vi "Debug - TCP - Log IP and Port.vi"(9 "IP and Port String":string, 10 "Flattened TCP Reference":string) -> ()   [LabVIEW 2017, in "Communications Library.lvlib"]
doc: "Edits the TCP debugging log file, so that the IP address and port are included in the contents.\n\nSaves changes to the file."
uses:
  Communications Library.lvlib
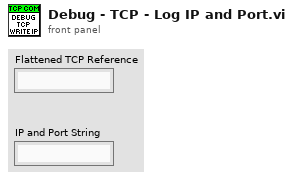
[diagram p1: front panel]
types:
  T1 = enum16{"open", "replace", "create", "open or create", "replace or create", "replace or create with confirmation"}
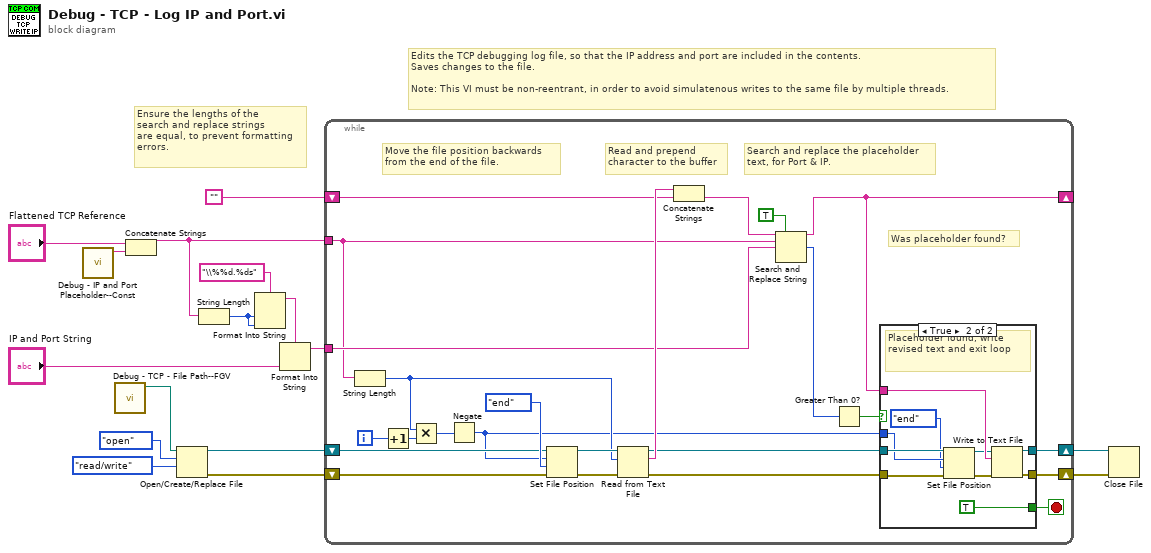
[diagram p0: block diagram]
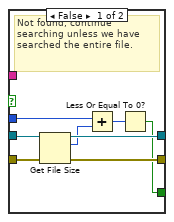
[diagram p2: hidden frame]
diagram:
  # "Ensure the lengths of the\nsearch and replace strings\nare equal, to prevent formatting\nerrors."
  # "Edits the TCP debugging log file, so that the IP address and port are included in the contents.\nSaves changes to the file.\n\nNote: This VI must be non-reentrant, in order to avoid simulatenous writes to the same file by multiple threads."
  n1 = call "Debug - IP and Port Placeholder--Const.vi"() -> ("Debug Placeholder"=w9:string)  [unwired: 11 in]
  n2 = call "Debug - TCP - File Path--FGV.vi"() -> ("Debug Pathname"=w7:path)  [unwired: 11 in]
  n3 = Concatenate Strings("Flattened TCP Reference", w9) -> (w3:string)
  n4 = Open/Create/Replace File(file path (use dialog)=w7, operation (0:open)=T1."open", access (0:read/write)=enum16{"read/write", "read-only", "write-only"}."read/write") -> (refnum out=w15:refnum<file>, error out=w16:errorcluster)  [unwired: 3 in, 1 out]
  n5 = String Length(string=w3) -> (length=w5:i32)
  n6 = Format Into String(format string="\\%%d.%ds", w5, w5) -> (resulting string=w6:string)  [unwired: 2 in, 1 out]
  n7 = Format Into String(format string=w6, "IP and Port String") -> (resulting string=w1:string)  [unwired: 2 in, 1 out]
  n8 = while {
    shift-right: [w18] -> _
    shift-left: "" -> [w30]
    tunnel: w3 -> [w17]
    tunnel: w1 -> [w28]
    shift-right: [w23] -> w10
    shift-left: w15 -> [w38]
    shift-right: [w22] -> w11
    shift-left: w16 -> [w39]
    i -> [w37]
    stop <- w21 stop-if-true
    # "Was placeholder found?"
    # "Search and replace the placeholder \ntext, for Port & IP."
    # "Read and prepend\ncharacter to the buffer"
    # "Move the file position backwards\nfrom the end of the file."
    n9 = String Length(string=w17) -> (length=w32:i32)
    n10 = Increment(x=w37) -> (x+1=w36:i32)
    n11 = Multiply(x=w32, y=w36) -> (x*y=w35:i32)
    n12 = Negate(x=w35) -> (-x=w20:i32)
    n13 = Set File Position(offset (in bytes) (0)=w20, refnum=w38, from (0:start)=enum16{"start", "end", "current"}."end", error in=w39) -> (refnum out=w34:refnum<file>, error out=w33:errorcluster)
    n14 = Read from Text File(file (use dialog)=w34, count=w32, error in=w33) -> (refnum out=w24:refnum<file>, text=w31:string, error out=w25:errorcluster)  [unwired: 1 in, 1 out]
    n15 = Concatenate Strings(w31, w30) -> (w19:string)
    n16 = Search and Replace String(replace all?=TRUE ("replace all? (F)"), input string=w19, search string=w17, replace string=w28) -> (result string=w18:string, number of replacements=w27:i32)  [unwired: 4 in, 2 out]
    n17 = Greater Than 0?(x=w27) -> (x > 0?=w26:bool)
    n18 = case shown="True" w26 {
      tunnel: w18 -> [_ w58]
      tunnel: w25 -> [w48 w54]
      tunnel: w24 -> [w47 w51]
      tunnel: [w46 w57] -> w23
      tunnel: [w45 w56] -> w22
      tunnel: [w41 TRUE] -> w21
      tunnel: w20 -> [w43 w50]
      frame False {
        # "Not found, continue\nsearching unless we have\nsearched the entire file."
        n19 = Get File Size(file=w47, error in=w48) -> (refnum out=w46:refnum<file>, size (in bytes)=w42:i64, 0:w45:errorcluster)
        n20 = Add(x=w43, y=w42) -> (x+y=w44:i64)
        n21 = Less Or Equal To 0?(x=w44) -> (x <= 0?=w41:bool)
      }
      frame True {
        # "Placeholder found, write\nrevised text and exit loop"
        n22 = Set File Position(offset (in bytes) (0)=w50, refnum=w51, from (0:start)=enum16{"start", "end", "current"}."end", error in=w54) -> (refnum out=w52:refnum<file>, error out=w53:errorcluster)
        n23 = Write to Text File(file (use dialog)=w52, text=w58, error in=w53) -> (refnum out=w57:refnum<file>, error out=w56:errorcluster)  [unwired: 1 in, 1 out]
      }
    }
  }
  n24 = Close File(refnum=w10, error in=w11) -> ()  [unwired: 2 out]
